vi "Inverse Chebyshev Filter PtByPt.vi"(4 "order":i32=2, 5 "initialize":bool, 6 "attenuation (dB)":dbl=60.0 format="%0.2f", 7 "filter type":T1, 8 "low cutoff freq: fl":dbl=0.125 format="%0.3f", 9 "high cutoff freq: fh":dbl=0.45000000000000007 format="%0.3f", 10 "sampling freq: fs":dbl=1.0 format="%0.2f", 11 "x":dbl format="%0.2f") -> (0 "error":i32, 3 "Filtered x":dbl format="%0.2f")   [LabVIEW 2020, in "NI_PtbyPt.lvlib"]
doc: "Generates a digital Chebyshev II filter using the Inv Chebyshev Coefficients algorithm."
uses:
  <vilib>/ptbypt/NI_PtbyPt.lvlib
  <vilib>/Analysis/3filter.llb/Filter Passband Type.ctl
  <vilib>/Analysis/NI_AALBase.lvlib
panel:
  # "PbP_Butterworth Filter"
  # "Filter Controls"
  # "Frequency Controls"
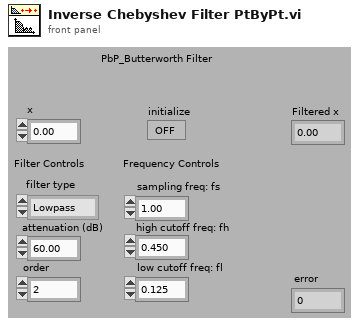
[diagram p1: front panel]
types:
  T1 = typedef "NI_AALBase.lvlib/Filter Passband Type.ctl" = enum32{"Lowpass", "Highpass", "Bandpass", "Bandstop"}
  T2 = cluster{"filter structure":enum32{"IIR 2nd Order", "IIR 4th Order"}, "Reverse Coefficients":dbl[], "Forward Coefficients":dbl[]}
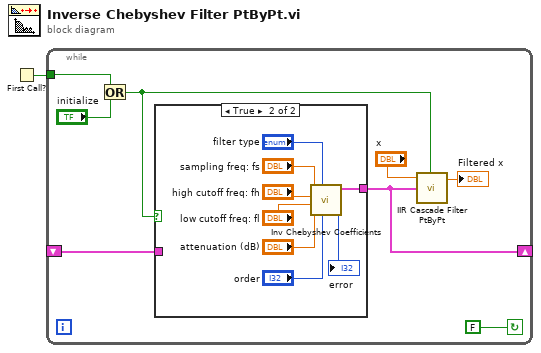
[diagram p0: block diagram]
diagram:
  n1 = First Call?() -> (First Call?: T/F=w1:bool)
  n2 = while {
    tunnel: w1 -> [w3]
    shift-left: _ -> [w8]
    shift-right: [w7] -> _
    stop <- FALSE continue-if-true
    n3 = Or(x=w3, y="initialize") -> (x .or. y?=w2:bool)
    n4 = case shown="True" w2 {
      tunnel: [w10 w18] -> w7
      tunnel: w8 -> [w10 _]
      frame False {
      }
      frame True {
        n5 = call <vilib>:"Inv Chebyshev Coefficients.vi"("order"="order", "filter type"="filter type", "attenuation (dB)"="attenuation (dB)", "low cutoff freq: fl"="low cutoff freq: fl", "high cutoff freq: fh"="high cutoff freq: fh", "sampling freq: fs"="sampling freq: fs") -> ("error"=→"error":i32, "IIR Filter Cluster"=w18:T2)  [unwired: 4 in]
      }
    }
    n6 = call <vilib>:"IIR Cascade Filter PtByPt.vi"("initialize"=w2, "IIR Filter Cluster"=w7, "x"="x") -> ("Filtered x"=→"Filtered x":dbl)  [unwired: 2 out]
  }
